vi "Global.vi"() -> ()   [LabVIEW 2020]
panel:
  in  "判定参数":T1
  out "数组":refnum<vi>[](array[refnum])
  in  "滑移力复检曲线":refnum<vi>
  in  "拉轴报表":refnum<vi>
  in  "滑移力报表":refnum<vi>
  in  "合格数量":i32
  in  "生产数量":i32
  in  "试验项目":bool[](array[boolean])
  out "模式":u32
  in  "更换产品":refnum<vi>
  in  "提示信息":refnum<vi>
  in  "程序自动":refnum<vi>
  in  "报警图标":refnum<vi>
  in  "程序关闭":bool
  in  "Info":refnum<vi>
  in  "Result":refnum<vi>
  in  "批次":refnum<vi>
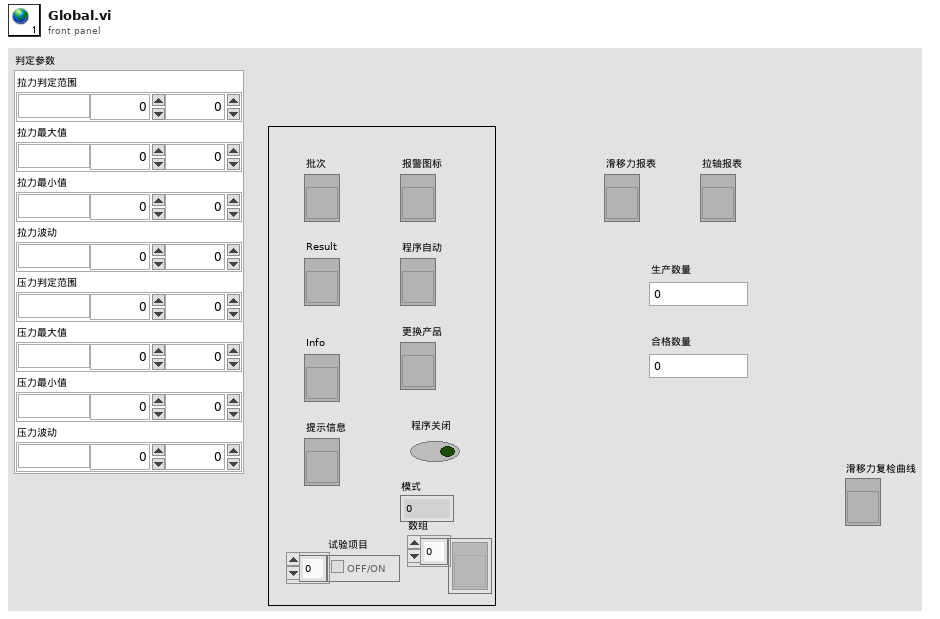
[diagram p1: front panel]
types:
  T1 = cluster{"拉力判定范围":cluster{"单位":string, "下限":dbl, "上限":dbl}, "拉力最大值":cluster{"单位":string, "下限":dbl, "上限":dbl}, "拉力最小值":cluster{"单位":string, "下限":dbl, "上限":dbl}, "拉力波动":cluster{"单位":string, "下限":dbl, "上限":dbl}, "压力判定范围":cluster{"单位":string, "下限":dbl, "上限":dbl}, "压力最大值":cluster{"单位":string, "下限":dbl, "上限":dbl}, "压力最小值":cluster{"单位":string, "下限":dbl, "上限":dbl}, "压力波动":cluster{"单位":string, "下限":dbl, "上限":dbl}}
diagram:
